vi "TCP-Generic Grab Data.vi"(0 "connection ID":refnum<k5>, 7 "No timeout?":bool, 11 "error in (no error)":errorcluster) -> (4 "connection ID out":refnum<k5>, 6 "data out":string, 15 "error out":errorcluster)   [LabVIEW 2020]
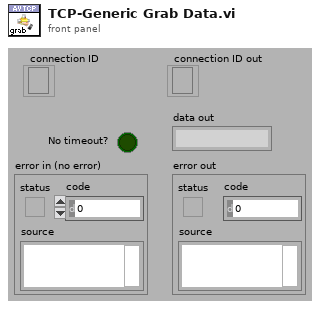
[diagram p1: front panel]
types:
  T1 = enum16{"big-endian, network order", "native, host order", "little-endian"}
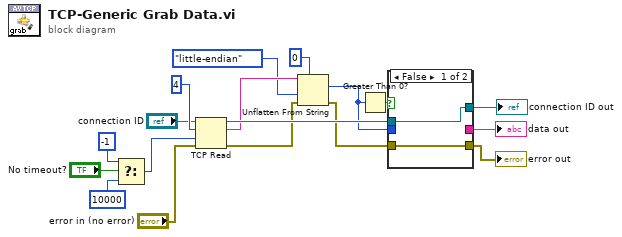
[diagram p0: block diagram]
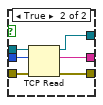
[diagram p2: hidden frame]
diagram:
  n1 = Select(t=-1 ("timeout ms (25000)"), s="No timeout?", f=10000 ("timeout ms (25000)")) -> (s? t:f=w10:i32)
  n2 = TCP Read(connection ID="connection ID", bytes to read=4, error in (no error)="error in (no error)", 9:w10) -> (connection ID out=w15:refnum<k5>, data out=w6:string, error out=w3:errorcluster)  [unwired: 1 in]
  n3 = Unflatten From String(type=0, binary string=w6, byte order (0:big-endian, network order)=T1."little-endian", error in (no error)=w3) -> (value=w2:i32, error out=w1:errorcluster)  [unwired: 1 in, 1 out]
  n4 = Greater Than 0?(x=w2) -> (x > 0?=w13:bool)
  n5 = case shown="False" w13 {
    tunnel: [_ w26] -> w18
    tunnel: [w20 w25] -> w17
    tunnel: w15 -> [w19 w24]
    tunnel: w1 -> [w20 w23]
    tunnel: w2 -> [_ w22]
    tunnel: [w19 w21] -> w7
    frame False {
    }
    frame True {
      n6 = TCP Read(connection ID=w24, bytes to read=w22, error in (no error)=w23) -> (connection ID out=w21:refnum<k5>, data out=w26:string, error out=w25:errorcluster)  [unwired: 2 in]
    }
  }
  "data out" <- w18
  "error out" <- w17
  "connection ID out" <- w7
